vi "Read Register (U16).vi"(0 "SLSC Interface in":refnum<class "SLSC Interface.lvclass">, 5 "device":refnum<k21>="$DefaultDevices", 7 "register address":u32 format="%.0x", 11 "error in (no error)":errorcluster) -> (4 "SLSC Interface out":refnum<class "SLSC Interface.lvclass">, 6 "device out":refnum<k21>, 8 "next register address":u32 format="%.0x", 10 "data out":u16 format="%.0x", 15 "error out":errorcluster)   [LabVIEW 2016, in "SLSC Interface.lvclass"]
uses:
  SLSC Interface.lvclass
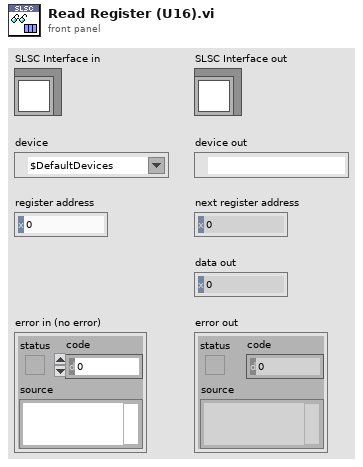
[diagram p1: front panel]
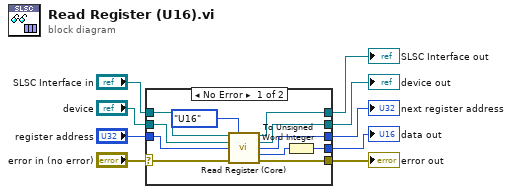
[diagram p0: block diagram]
diagram:
  n1 = case shown="No Error" "error in (no error)" {
    selector: "error in (no error)" -> [w18 w24]
    tunnel: [w17 w24] -> w8
    tunnel: [w19 w23] -> w6
    tunnel: "SLSC Interface in" -> [w20 w23]
    tunnel: "register address" -> [w12 w22]
    tunnel: [w15 w21] -> w4
    tunnel: [w14 w22] -> w3
    tunnel: [w10 _] -> w2
    tunnel: "device" -> [w13 w21]
    frame No Error {
      n2 = call "Read Register (Core).vi"("SLSC Interface in"=w20, "type"=enum16{"U8", "U16", "U32", "U64"}."U16" ("size"), "device"=w13, "register address"=w12, "error in (no error)"=w18) -> ("SLSC Interface out"=w19:refnum<class "SLSC Interface.lvclass">, "device out"=w15:refnum<k21>, "next register address"=w14:u32, "data out"=w11:u64, "error out"=w17:errorcluster)  [unwired: 6 in]
      n3 = To Unsigned Word Integer(number=w11) -> (unsigned 16bit integer=w10:u16)
    }
    frame Error {
    }
  }
  "error out" <- w8
  "SLSC Interface out" <- w6
  "device out" <- w4
  "next register address" <- w3
  "data out" <- w2
